vi "Filter And List Controls.vi"(8 "Error In":errorcluster, 10 "Control Refs":refnum<vi>[](array[refnum]), 11 "Control Reference Lists In":T1) -> (0 "Error Out":errorcluster, 3 "Control Reference Lists Out":T1)   [LabVIEW 2021, in "Appearance Actor.lvlib" / "Appearance Actor.lvclass"]
uses:
  Appearance Actor.lvclass
  Typedefs/Control Reference Lists--cluster.ctl
  Typedefs/Control Reference Lists-TitleBar--cluster.ctl
  Typedefs/Control Reference Lists-SideMenu--cluster.ctl
  Typedefs/Control Reference Lists-BodyPane--cluster.ctl
  Typedefs/Control Reference Lists-StatusBar--cluster.ctl
  <vilib>/regexp/Match Regular Expression.xnode
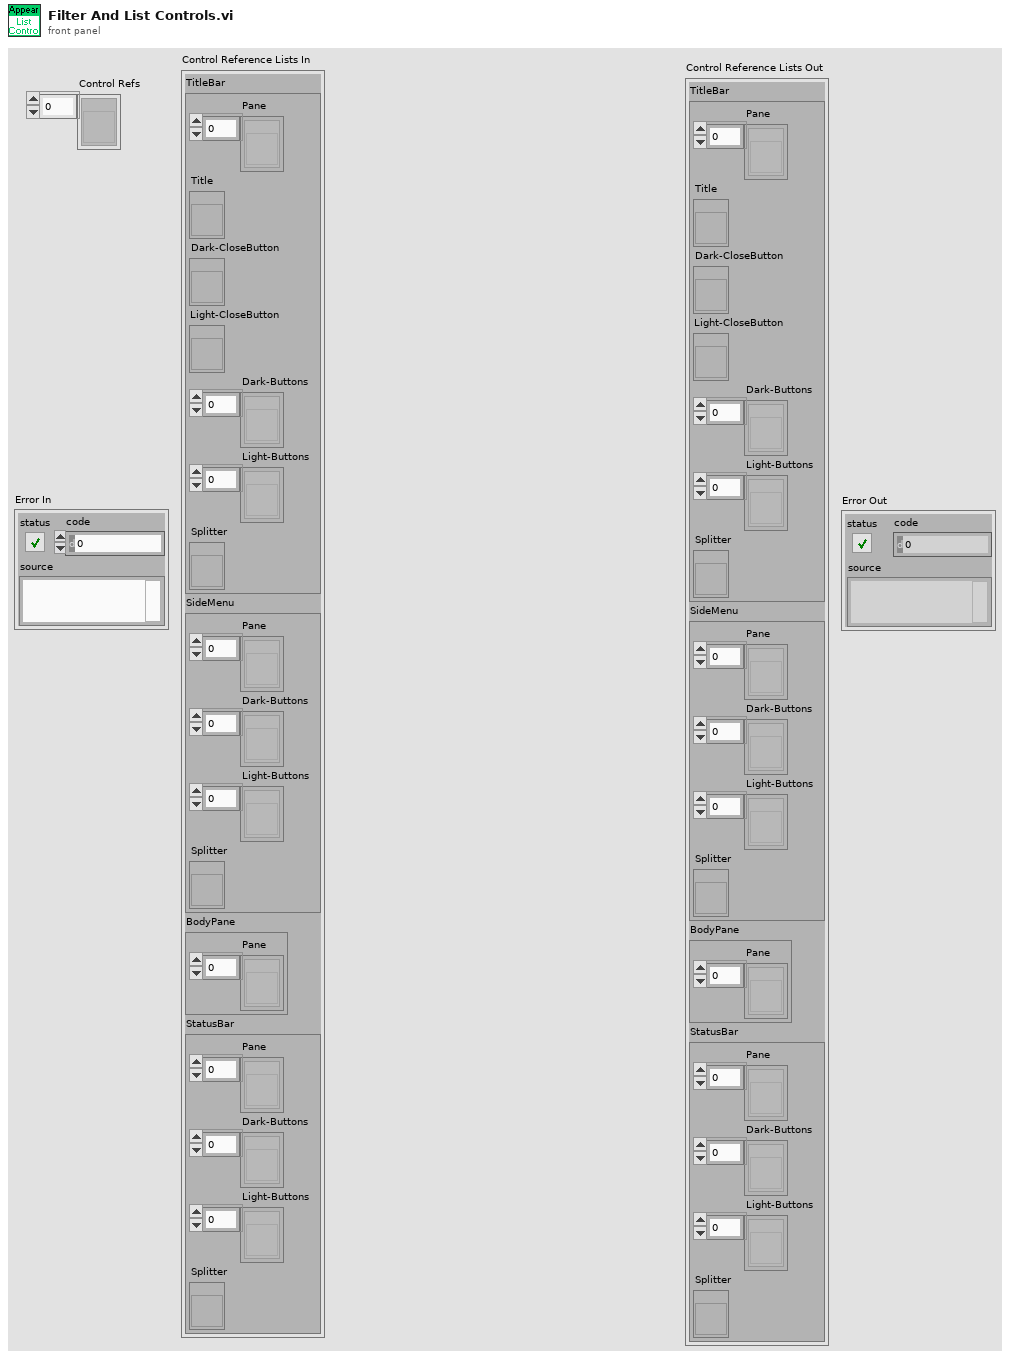
[diagram p1: front panel]
types:
  T1 = typedef "Appearance Actor.lvlib/Appearance Actor.lvclass/Control Reference Lists--cluster.ctl" = cluster{"TitleBar":T2, "SideMenu":T3, "BodyPane":T4, "StatusBar":T5}
  T2 = typedef "Appearance Actor.lvlib/Appearance Actor.lvclass/Control Reference Lists-TitleBar--cluster.ctl" = cluster{"Pane":refnum<vi>[], "Title":refnum<vi>, "Dark-CloseButton":refnum<vi>, "Light-CloseButton":refnum<vi>, "Dark-Buttons":refnum<vi>[], "Light-Buttons":refnum<vi>[], "Splitter":refnum<vi>}
  T3 = typedef "Appearance Actor.lvlib/Appearance Actor.lvclass/Control Reference Lists-SideMenu--cluster.ctl" = cluster{"Pane":refnum<vi>[], "Dark-Buttons":refnum<vi>[], "Light-Buttons":refnum<vi>[], "Splitter":refnum<vi>}
  T4 = typedef "Appearance Actor.lvlib/Appearance Actor.lvclass/Control Reference Lists-BodyPane--cluster.ctl" = cluster{"Pane":refnum<vi>[]}
  T5 = typedef "Appearance Actor.lvlib/Appearance Actor.lvclass/Control Reference Lists-StatusBar--cluster.ctl" = cluster{"Pane":refnum<vi>[], "Dark-Buttons":refnum<vi>[], "Light-Buttons":refnum<vi>[], "Splitter":refnum<vi>}
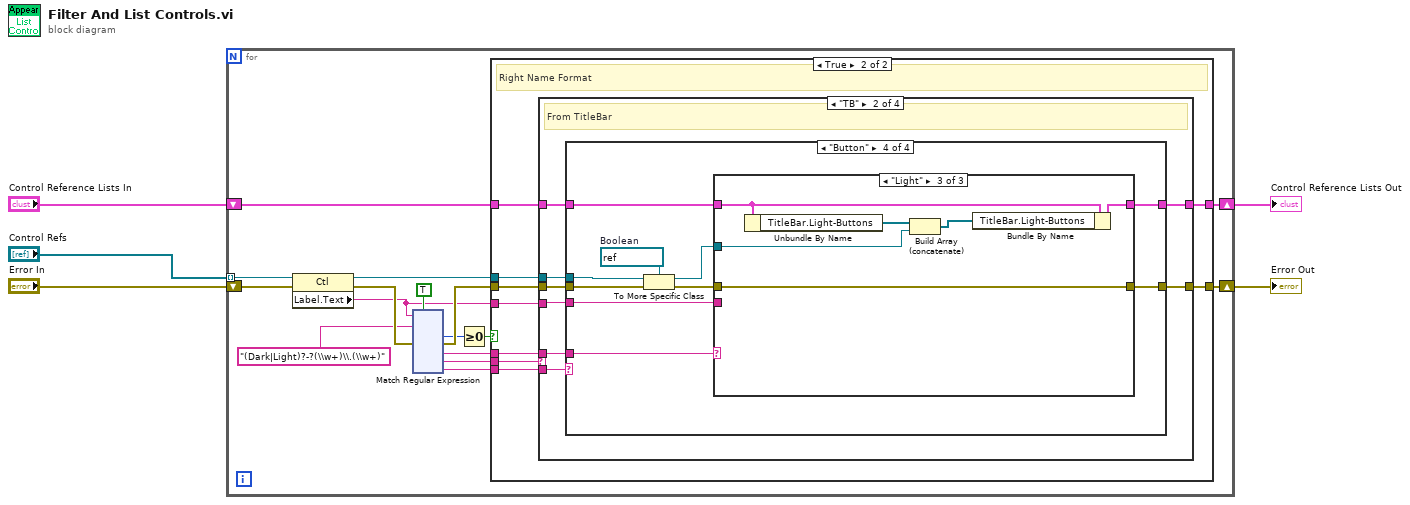
[diagram p0: block diagram]
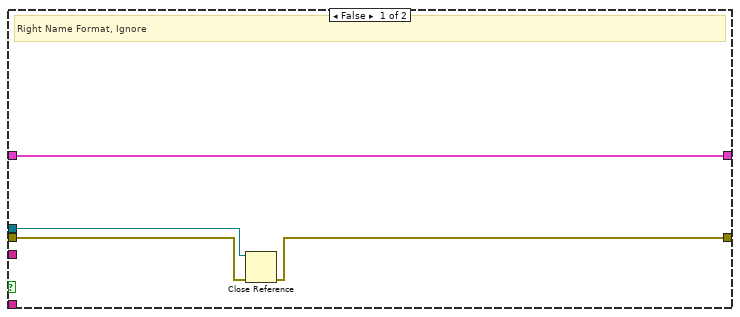
[diagram p2: hidden frame]
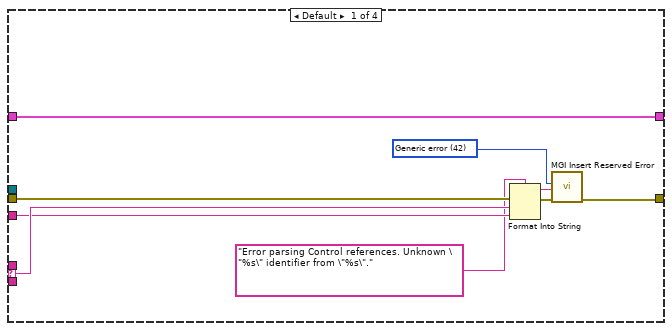
[diagram p3: hidden frame]
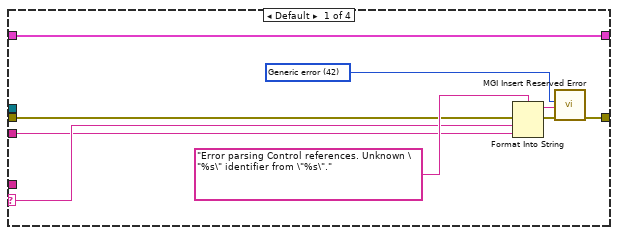
[diagram p4: hidden frame]
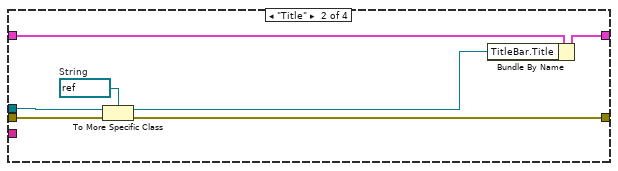
[diagram p5: hidden frame]
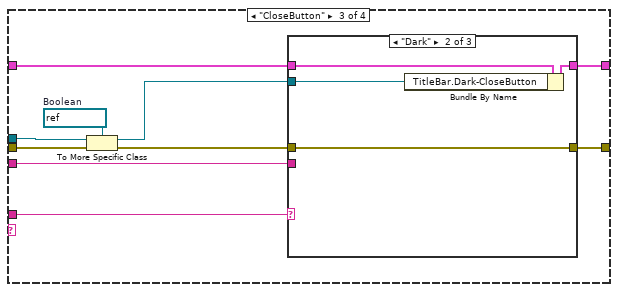
[diagram p6: hidden frame]
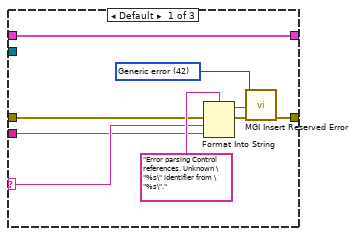
[diagram p7: hidden frame]
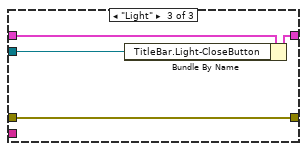
[diagram p8: hidden frame]
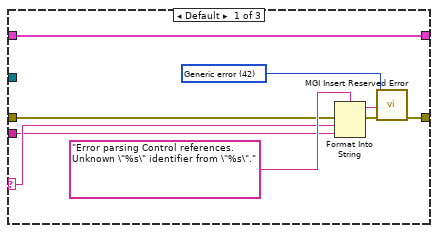
[diagram p9: hidden frame]
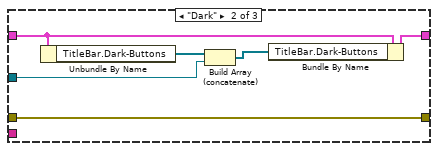
[diagram p10: hidden frame]
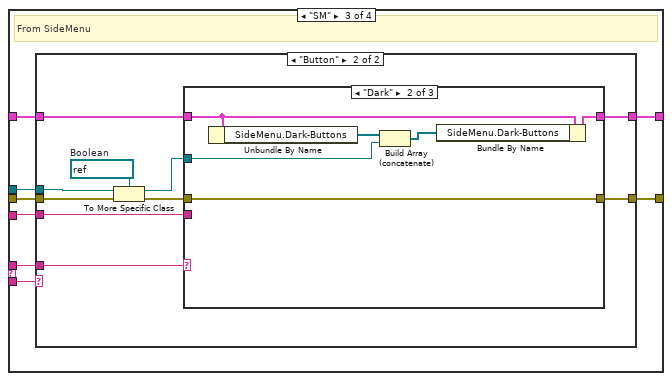
[diagram p11: hidden frame]
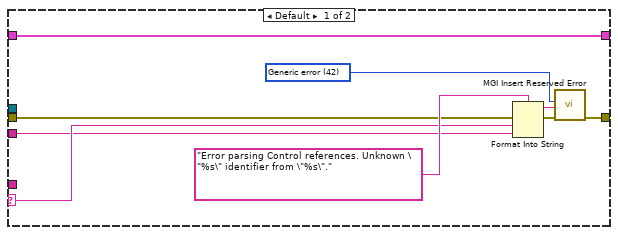
[diagram p12: hidden frame]
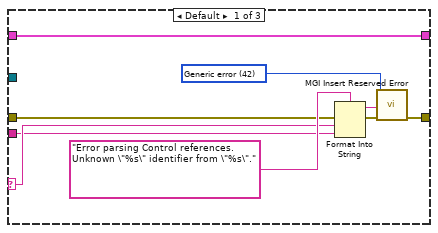
[diagram p13: hidden frame]
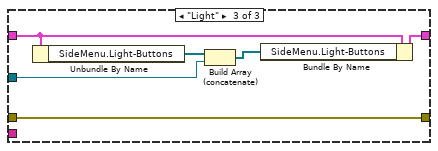
[diagram p14: hidden frame]
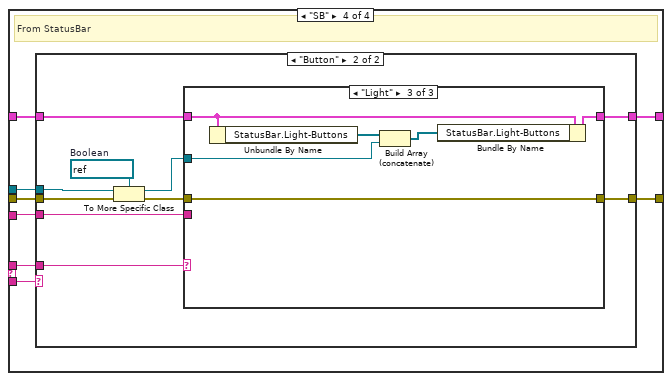
[diagram p15: hidden frame]
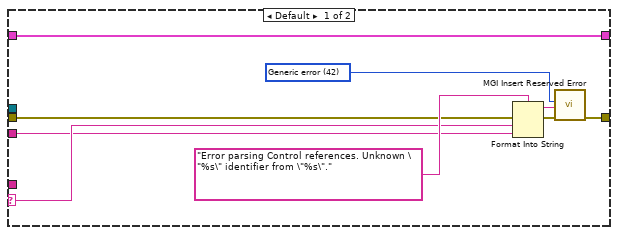
[diagram p16: hidden frame]
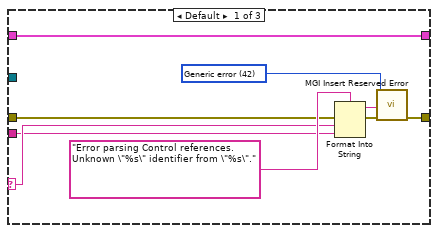
[diagram p17: hidden frame]
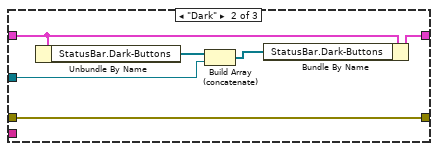
[diagram p18: hidden frame]
diagram:
  n1 = for {
    shift-right: [w9] -> w4
    shift-left: "Control Reference Lists In" -> [w16]
    shift-right: [w14] -> w3
    shift-left: "Error In" -> [w20]
    tunnel: "Control Refs" -> [w21] mode=indexing
    n2 = property class="Ctl"(reference=w21, error in=w20) -> (reference out=w8:refnum<vi>, error out=w19:errorcluster, "Label.Text"=w10:string)
    n3 = xnode "Match Regular Expression"("input string"=w10, "regular expression"="(Dark|Light)?-?(\\w+)\\.(\\w+)", "error in"=w19, "ignore case? (F)"=TRUE) -> ("offset past match"=w7:i32, "error out"=w13:errorcluster, "submatch 1"=w12:string, "submatch 2"=w15:string, "submatch 3"=w11:string)  [unwired: 2 in, 3 out]
    n4 = Greater Or Equal To 0?(x=w7) -> (x >= 0?=w6:bool)
    n5 = case shown="True" w6 {
      tunnel: w16 -> [w25 w34]
      tunnel: w15 -> [_ w33]
      tunnel: [w22 w32] -> w14
      tunnel: w13 -> [w23 w31]
      tunnel: w12 -> [_ w30]
      tunnel: w11 -> [_ w29]
      tunnel: w10 -> [_ w28]
      tunnel: [w25 w27] -> w9
      tunnel: w8 -> [w24 w26]
      frame False {
        # "Right Name Format, Ignore"
        n6 = Close Reference(reference=w24, error in (no error)=w23) -> (error out=w22:errorcluster)
      }
      frame True {
        # "Right Name Format"
        n7 = case shown="\"TB\"" w33 {
          selector: w33 -> [w38 _ _ _]
          tunnel: w34 -> [w36 w47 w129 w177]
          tunnel: [w39 w49 w131 w179] -> w32
          tunnel: w31 -> [w40 w50 w132 w180]
          tunnel: w30 -> [_ w44 w126 w174]
          tunnel: w29 -> [_ w51 w133 w181]
          tunnel: w28 -> [w37 w48 w130 w178]
          tunnel: [w36 w46 w128 w176] -> w27
          tunnel: w26 -> [_ w45 w127 w175]
          frame Default {
            w41 = 42 items=["No error", "Argument error", "Memory is full", "Out of zone", "End of file", "File already open", "Generic file I/O error", "File not found", "File permission error", "Disk is full", "Duplicate path", "Too many files open", "System feature not enabled", "Resource file not found", "Cannot add resource", "Resource not found", "Image not found", "Image memory error", "Pen does not exist", "Config type invalid", "Config token not found", "Config parse error", "Config memory error", "Bad external code format", "Bad external code offset", "External code not present", "Null window", "Destroy window error", "Null menu", "Print aborted", "Bad print record", "Print driver error", "Windows error during printing", "Memory error during printing", "Print dialog error", "Generic print error", "Invalid device refnum", "Device not found", "Device parameter error", "Device unit error", "Cannot open device", "Device call aborted", "Generic error", "Cancelled by user", "Object ID too low", "Object ID too high", "Object not in heap", "Unknown heap", "Unknown object (invalid DefProc)", "Unknown object (DefProc not in table)", "Message out of range", "Invalid (null) method", "Unknown message", "Manager call not supported", "Bad address", "Network operation in progress", "Network operation timed out", "Connection is busy", "Network attribute not supported", "Network error", "Address in use", "System out of memory", "Connection aborted", "Connection refused", "Not connected", "Already connected", "Connection closed", "Initialization error (interapplication manager)", "Bad occurrence", "Wait on unbound occurrence handler", "Occurrence queue overflow", "Datalog type conflict", "Unused", "Unrecognized type (interapplication manager)", "Memory corrupt", "Failed to make temporary DLL", "Old CIN version", "Drag socket not found", "Failed to load drop-object", "Failed to register OLE object", "Failed to release OLE object", "Format specifier type mismatch", "Unknown format specifier", "Too few format specifiers", "Too many format specifiers", "Scan failed", "Newer CIN version", "OLE Convert", "Runtime menu error", "Password tampered", "Unknown error code"] ("Reserved Error Code (Generic error)")
            n8 = Format Into String(format string="Error parsing Control references. Unknown \"%s\" identifier from \"%s\".", error in=w40, w38, w37) -> (resulting string=w43:string, error out=w42:errorcluster)  [unwired: 1 in]
            n9 = call <userlib>:"MGI Insert Reserved Error.vi"("Error In"=w42, "Error Description"=w43, "Reserved Error Code (Generic error)"=w41) -> ("Error Out"=w39:errorcluster)  [unwired: 8 in]
          }
          frame "TB" {
            # "From TitleBar"
            n10 = case shown="\"Button\"" w51 {
              selector: w51 -> [w54 _ _ _]
              tunnel: w50 -> [w56 w62 w72 w99]
              tunnel: [w55 w61 w69 w96] -> w49
              tunnel: w48 -> [w53 _ w68 w95]
              tunnel: w47 -> [w52 w67 w77 w104]
              tunnel: [w52 w66 w76 w103] -> w46
              tunnel: w45 -> [_ w64 w74 w101]
              tunnel: w44 -> [_ _ w71 w98]
              frame Default {
                w58 = 42 items=["No error", "Argument error", "Memory is full", "Out of zone", "End of file", "File already open", "Generic file I/O error", "File not found", "File permission error", "Disk is full", "Duplicate path", "Too many files open", "System feature not enabled", "Resource file not found", "Cannot add resource", "Resource not found", "Image not found", "Image memory error", "Pen does not exist", "Config type invalid", "Config token not found", "Config parse error", "Config memory error", "Bad external code format", "Bad external code offset", "External code not present", "Null window", "Destroy window error", "Null menu", "Print aborted", "Bad print record", "Print driver error", "Windows error during printing", "Memory error during printing", "Print dialog error", "Generic print error", "Invalid device refnum", "Device not found", "Device parameter error", "Device unit error", "Cannot open device", "Device call aborted", "Generic error", "Cancelled by user", "Object ID too low", "Object ID too high", "Object not in heap", "Unknown heap", "Unknown object (invalid DefProc)", "Unknown object (DefProc not in table)", "Message out of range", "Invalid (null) method", "Unknown message", "Manager call not supported", "Bad address", "Network operation in progress", "Network operation timed out", "Connection is busy", "Network attribute not supported", "Network error", "Address in use", "System out of memory", "Connection aborted", "Connection refused", "Not connected", "Already connected", "Connection closed", "Initialization error (interapplication manager)", "Bad occurrence", "Wait on unbound occurrence handler", "Occurrence queue overflow", "Datalog type conflict", "Unused", "Unrecognized type (interapplication manager)", "Memory corrupt", "Failed to make temporary DLL", "Old CIN version", "Drag socket not found", "Failed to load drop-object", "Failed to register OLE object", "Failed to release OLE object", "Format specifier type mismatch", "Unknown format specifier", "Too few format specifiers", "Too many format specifiers", "Scan failed", "Newer CIN version", "OLE Convert", "Runtime menu error", "Password tampered", "Unknown error code"] ("Reserved Error Code (Generic error)")
                n11 = Format Into String(format string="Error parsing Control references. Unknown \"%s\" identifier from \"%s\".", error in=w56, w54, w53) -> (resulting string=w60:string, error out=w59:errorcluster)  [unwired: 1 in]
                n12 = call <userlib>:"MGI Insert Reserved Error.vi"("Error In"=w59, "Error Description"=w60, "Reserved Error Code (Generic error)"=w58) -> ("Error Out"=w55:errorcluster)  [unwired: 8 in]
              }
              frame "Title" {
                w65 = refnum<vi> refnum  # String
                n13 = To More Specific Class(target class=w65, reference=w64, error in=w62) -> (specific class reference=w63:refnum<vi>, error out=w61:errorcluster)
                n14 = Bundle By Name(cluster=w67, "TitleBar.Title"=w63) -> (w66:T1)
              }
              frame "CloseButton" {
                w75 = refnum<vi> refnum  # Boolean
                n15 = To More Specific Class(target class=w75, reference=w74, error in=w72) -> (specific class reference=w73:refnum<vi>, error out=w70:errorcluster)
                n16 = case shown="\"Dark\"" w71 {
                  selector: w71 -> [w79 _ _]
                  tunnel: w77 -> [w80 w90 w94]
                  tunnel: [w80 w89 w93] -> w76
                  tunnel: w73 -> [_ w88 w92]
                  tunnel: w70 -> [w82 w87 w91]
                  tunnel: [w81 w87 w91] -> w69
                  tunnel: w68 -> [w78 _ _]
                  frame Default {
                    w84 = 42 items=["No error", "Argument error", "Memory is full", "Out of zone", "End of file", "File already open", "Generic file I/O error", "File not found", "File permission error", "Disk is full", "Duplicate path", "Too many files open", "System feature not enabled", "Resource file not found", "Cannot add resource", "Resource not found", "Image not found", "Image memory error", "Pen does not exist", "Config type invalid", "Config token not found", "Config parse error", "Config memory error", "Bad external code format", "Bad external code offset", "External code not present", "Null window", "Destroy window error", "Null menu", "Print aborted", "Bad print record", "Print driver error", "Windows error during printing", "Memory error during printing", "Print dialog error", "Generic print error", "Invalid device refnum", "Device not found", "Device parameter error", "Device unit error", "Cannot open device", "Device call aborted", "Generic error", "Cancelled by user", "Object ID too low", "Object ID too high", "Object not in heap", "Unknown heap", "Unknown object (invalid DefProc)", "Unknown object (DefProc not in table)", "Message out of range", "Invalid (null) method", "Unknown message", "Manager call not supported", "Bad address", "Network operation in progress", "Network operation timed out", "Connection is busy", "Network attribute not supported", "Network error", "Address in use", "System out of memory", "Connection aborted", "Connection refused", "Not connected", "Already connected", "Connection closed", "Initialization error (interapplication manager)", "Bad occurrence", "Wait on unbound occurrence handler", "Occurrence queue overflow", "Datalog type conflict", "Unused", "Unrecognized type (interapplication manager)", "Memory corrupt", "Failed to make temporary DLL", "Old CIN version", "Drag socket not found", "Failed to load drop-object", "Failed to register OLE object", "Failed to release OLE object", "Format specifier type mismatch", "Unknown format specifier", "Too few format specifiers", "Too many format specifiers", "Scan failed", "Newer CIN version", "OLE Convert", "Runtime menu error", "Password tampered", "Unknown error code"] ("Reserved Error Code (Generic error)")
                    n17 = Format Into String(format string="Error parsing Control references. Unknown \"%s\" identifier from \"%s\".", error in=w82, w79, w78) -> (resulting string=w86:string, error out=w85:errorcluster)  [unwired: 1 in]
                    n18 = call <userlib>:"MGI Insert Reserved Error.vi"("Error In"=w85, "Error Description"=w86, "Reserved Error Code (Generic error)"=w84) -> ("Error Out"=w81:errorcluster)  [unwired: 8 in]
                  }
                  frame "Dark" {
                    n19 = Bundle By Name(cluster=w90, "TitleBar.Dark-CloseButton"=w88) -> (w89:T1)
                  }
                  frame "Light" {
                    n20 = Bundle By Name(cluster=w94, "TitleBar.Light-CloseButton"=w92) -> (w93:T1)
                  }
                }
              }
              frame "Button" {
                w102 = refnum<vi> refnum  # Boolean
                n21 = To More Specific Class(target class=w102, reference=w101, error in=w99) -> (specific class reference=w100:refnum<vi>, error out=w97:errorcluster)
                n22 = case shown="\"Light\"" w98 {
                  selector: w98 -> [w106 _ _]
                  tunnel: w104 -> [w107 w117 w123]
                  tunnel: [w107 w119 w125] -> w103
                  tunnel: w100 -> [_ w114 w120]
                  tunnel: w97 -> [w109 w118 w124]
                  tunnel: [w108 w118 w124] -> w96
                  tunnel: w95 -> [w105 _ _]
                  frame Default {
                    w111 = 42 items=["No error", "Argument error", "Memory is full", "Out of zone", "End of file", "File already open", "Generic file I/O error", "File not found", "File permission error", "Disk is full", "Duplicate path", "Too many files open", "System feature not enabled", "Resource file not found", "Cannot add resource", "Resource not found", "Image not found", "Image memory error", "Pen does not exist", "Config type invalid", "Config token not found", "Config parse error", "Config memory error", "Bad external code format", "Bad external code offset", "External code not present", "Null window", "Destroy window error", "Null menu", "Print aborted", "Bad print record", "Print driver error", "Windows error during printing", "Memory error during printing", "Print dialog error", "Generic print error", "Invalid device refnum", "Device not found", "Device parameter error", "Device unit error", "Cannot open device", "Device call aborted", "Generic error", "Cancelled by user", "Object ID too low", "Object ID too high", "Object not in heap", "Unknown heap", "Unknown object (invalid DefProc)", "Unknown object (DefProc not in table)", "Message out of range", "Invalid (null) method", "Unknown message", "Manager call not supported", "Bad address", "Network operation in progress", "Network operation timed out", "Connection is busy", "Network attribute not supported", "Network error", "Address in use", "System out of memory", "Connection aborted", "Connection refused", "Not connected", "Already connected", "Connection closed", "Initialization error (interapplication manager)", "Bad occurrence", "Wait on unbound occurrence handler", "Occurrence queue overflow", "Datalog type conflict", "Unused", "Unrecognized type (interapplication manager)", "Memory corrupt", "Failed to make temporary DLL", "Old CIN version", "Drag socket not found", "Failed to load drop-object", "Failed to register OLE object", "Failed to release OLE object", "Format specifier type mismatch", "Unknown format specifier", "Too few format specifiers", "Too many format specifiers", "Scan failed", "Newer CIN version", "OLE Convert", "Runtime menu error", "Password tampered", "Unknown error code"] ("Reserved Error Code (Generic error)")
                    n23 = Format Into String(format string="Error parsing Control references. Unknown \"%s\" identifier from \"%s\".", error in=w109, w106, w105) -> (resulting string=w113:string, error out=w112:errorcluster)  [unwired: 1 in]
                    n24 = call <userlib>:"MGI Insert Reserved Error.vi"("Error In"=w112, "Error Description"=w113, "Reserved Error Code (Generic error)"=w111) -> ("Error Out"=w108:errorcluster)  [unwired: 8 in]
                  }
                  frame "Dark" {
                    n25 = Unbundle By Name(w117) -> ("TitleBar.Dark-Buttons"=w116:refnum<vi>[])
                    n26 = Build Array (concatenate)(w116, w114) -> (w115:refnum<vi>[])
                    n27 = Bundle By Name(cluster=w117, "TitleBar.Dark-Buttons"=w115) -> (w119:T1)
                  }
                  frame "Light" {
                    n28 = Unbundle By Name(w123) -> ("TitleBar.Light-Buttons"=w122:refnum<vi>[])
                    n29 = Build Array (concatenate)(w122, w120) -> (w121:refnum<vi>[])
                    n30 = Bundle By Name(cluster=w123, "TitleBar.Light-Buttons"=w121) -> (w125:T1)
                  }
                }
              }
            }
          }
          frame "SM" {
            # "From SideMenu"
            n31 = case shown="\"Button\"" w133 {
              selector: w133 -> [w136 _]
              tunnel: w132 -> [w138 w147]
              tunnel: [w137 w144] -> w131
              tunnel: w130 -> [w135 w143]
              tunnel: w129 -> [w134 w152]
              tunnel: [w134 w151] -> w128
              tunnel: w127 -> [_ w149]
              tunnel: w126 -> [_ w146]
              frame Default {
                w140 = 42 items=["No error", "Argument error", "Memory is full", "Out of zone", "End of file", "File already open", "Generic file I/O error", "File not found", "File permission error", "Disk is full", "Duplicate path", "Too many files open", "System feature not enabled", "Resource file not found", "Cannot add resource", "Resource not found", "Image not found", "Image memory error", "Pen does not exist", "Config type invalid", "Config token not found", "Config parse error", "Config memory error", "Bad external code format", "Bad external code offset", "External code not present", "Null window", "Destroy window error", "Null menu", "Print aborted", "Bad print record", "Print driver error", "Windows error during printing", "Memory error during printing", "Print dialog error", "Generic print error", "Invalid device refnum", "Device not found", "Device parameter error", "Device unit error", "Cannot open device", "Device call aborted", "Generic error", "Cancelled by user", "Object ID too low", "Object ID too high", "Object not in heap", "Unknown heap", "Unknown object (invalid DefProc)", "Unknown object (DefProc not in table)", "Message out of range", "Invalid (null) method", "Unknown message", "Manager call not supported", "Bad address", "Network operation in progress", "Network operation timed out", "Connection is busy", "Network attribute not supported", "Network error", "Address in use", "System out of memory", "Connection aborted", "Connection refused", "Not connected", "Already connected", "Connection closed", "Initialization error (interapplication manager)", "Bad occurrence", "Wait on unbound occurrence handler", "Occurrence queue overflow", "Datalog type conflict", "Unused", "Unrecognized type (interapplication manager)", "Memory corrupt", "Failed to make temporary DLL", "Old CIN version", "Drag socket not found", "Failed to load drop-object", "Failed to register OLE object", "Failed to release OLE object", "Format specifier type mismatch", "Unknown format specifier", "Too few format specifiers", "Too many format specifiers", "Scan failed", "Newer CIN version", "OLE Convert", "Runtime menu error", "Password tampered", "Unknown error code"] ("Reserved Error Code (Generic error)")
                n32 = Format Into String(format string="Error parsing Control references. Unknown \"%s\" identifier from \"%s\".", error in=w138, w136, w135) -> (resulting string=w142:string, error out=w141:errorcluster)  [unwired: 1 in]
                n33 = call <userlib>:"MGI Insert Reserved Error.vi"("Error In"=w141, "Error Description"=w142, "Reserved Error Code (Generic error)"=w140) -> ("Error Out"=w137:errorcluster)  [unwired: 8 in]
              }
              frame "Button" {
                w150 = refnum<vi> refnum  # Boolean
                n34 = To More Specific Class(target class=w150, reference=w149, error in=w147) -> (specific class reference=w148:refnum<vi>, error out=w145:errorcluster)
                n35 = case shown="\"Dark\"" w146 {
                  selector: w146 -> [w154 _ _]
                  tunnel: w152 -> [w155 w165 w171]
                  tunnel: [w155 w167 w173] -> w151
                  tunnel: w148 -> [_ w162 w168]
                  tunnel: w145 -> [w157 w166 w172]
                  tunnel: [w156 w166 w172] -> w144
                  tunnel: w143 -> [w153 _ _]
                  frame Default {
                    w159 = 42 items=["No error", "Argument error", "Memory is full", "Out of zone", "End of file", "File already open", "Generic file I/O error", "File not found", "File permission error", "Disk is full", "Duplicate path", "Too many files open", "System feature not enabled", "Resource file not found", "Cannot add resource", "Resource not found", "Image not found", "Image memory error", "Pen does not exist", "Config type invalid", "Config token not found", "Config parse error", "Config memory error", "Bad external code format", "Bad external code offset", "External code not present", "Null window", "Destroy window error", "Null menu", "Print aborted", "Bad print record", "Print driver error", "Windows error during printing", "Memory error during printing", "Print dialog error", "Generic print error", "Invalid device refnum", "Device not found", "Device parameter error", "Device unit error", "Cannot open device", "Device call aborted", "Generic error", "Cancelled by user", "Object ID too low", "Object ID too high", "Object not in heap", "Unknown heap", "Unknown object (invalid DefProc)", "Unknown object (DefProc not in table)", "Message out of range", "Invalid (null) method", "Unknown message", "Manager call not supported", "Bad address", "Network operation in progress", "Network operation timed out", "Connection is busy", "Network attribute not supported", "Network error", "Address in use", "System out of memory", "Connection aborted", "Connection refused", "Not connected", "Already connected", "Connection closed", "Initialization error (interapplication manager)", "Bad occurrence", "Wait on unbound occurrence handler", "Occurrence queue overflow", "Datalog type conflict", "Unused", "Unrecognized type (interapplication manager)", "Memory corrupt", "Failed to make temporary DLL", "Old CIN version", "Drag socket not found", "Failed to load drop-object", "Failed to register OLE object", "Failed to release OLE object", "Format specifier type mismatch", "Unknown format specifier", "Too few format specifiers", "Too many format specifiers", "Scan failed", "Newer CIN version", "OLE Convert", "Runtime menu error", "Password tampered", "Unknown error code"] ("Reserved Error Code (Generic error)")
                    n36 = Format Into String(format string="Error parsing Control references. Unknown \"%s\" identifier from \"%s\".", error in=w157, w154, w153) -> (resulting string=w161:string, error out=w160:errorcluster)  [unwired: 1 in]
                    n37 = call <userlib>:"MGI Insert Reserved Error.vi"("Error In"=w160, "Error Description"=w161, "Reserved Error Code (Generic error)"=w159) -> ("Error Out"=w156:errorcluster)  [unwired: 8 in]
                  }
                  frame "Dark" {
                    n38 = Unbundle By Name(w165) -> ("SideMenu.Dark-Buttons"=w164:refnum<vi>[])
                    n39 = Build Array (concatenate)(w164, w162) -> (w163:refnum<vi>[])
                    n40 = Bundle By Name(cluster=w165, "SideMenu.Dark-Buttons"=w163) -> (w167:T1)
                  }
                  frame "Light" {
                    n41 = Unbundle By Name(w171) -> ("SideMenu.Light-Buttons"=w170:refnum<vi>[])
                    n42 = Build Array (concatenate)(w170, w168) -> (w169:refnum<vi>[])
                    n43 = Bundle By Name(cluster=w171, "SideMenu.Light-Buttons"=w169) -> (w173:T1)
                  }
                }
              }
            }
          }
          frame "SB" {
            # "From StatusBar"
            n44 = case shown="\"Button\"" w181 {
              selector: w181 -> [w184 _]
              tunnel: w180 -> [w186 w195]
              tunnel: [w185 w192] -> w179
              tunnel: w178 -> [w183 w191]
              tunnel: w177 -> [w182 w200]
              tunnel: [w182 w199] -> w176
              tunnel: w175 -> [_ w197]
              tunnel: w174 -> [_ w194]
              frame Default {
                w188 = 42 items=["No error", "Argument error", "Memory is full", "Out of zone", "End of file", "File already open", "Generic file I/O error", "File not found", "File permission error", "Disk is full", "Duplicate path", "Too many files open", "System feature not enabled", "Resource file not found", "Cannot add resource", "Resource not found", "Image not found", "Image memory error", "Pen does not exist", "Config type invalid", "Config token not found", "Config parse error", "Config memory error", "Bad external code format", "Bad external code offset", "External code not present", "Null window", "Destroy window error", "Null menu", "Print aborted", "Bad print record", "Print driver error", "Windows error during printing", "Memory error during printing", "Print dialog error", "Generic print error", "Invalid device refnum", "Device not found", "Device parameter error", "Device unit error", "Cannot open device", "Device call aborted", "Generic error", "Cancelled by user", "Object ID too low", "Object ID too high", "Object not in heap", "Unknown heap", "Unknown object (invalid DefProc)", "Unknown object (DefProc not in table)", "Message out of range", "Invalid (null) method", "Unknown message", "Manager call not supported", "Bad address", "Network operation in progress", "Network operation timed out", "Connection is busy", "Network attribute not supported", "Network error", "Address in use", "System out of memory", "Connection aborted", "Connection refused", "Not connected", "Already connected", "Connection closed", "Initialization error (interapplication manager)", "Bad occurrence", "Wait on unbound occurrence handler", "Occurrence queue overflow", "Datalog type conflict", "Unused", "Unrecognized type (interapplication manager)", "Memory corrupt", "Failed to make temporary DLL", "Old CIN version", "Drag socket not found", "Failed to load drop-object", "Failed to register OLE object", "Failed to release OLE object", "Format specifier type mismatch", "Unknown format specifier", "Too few format specifiers", "Too many format specifiers", "Scan failed", "Newer CIN version", "OLE Convert", "Runtime menu error", "Password tampered", "Unknown error code"] ("Reserved Error Code (Generic error)")
                n45 = Format Into String(format string="Error parsing Control references. Unknown \"%s\" identifier from \"%s\".", error in=w186, w184, w183) -> (resulting string=w190:string, error out=w189:errorcluster)  [unwired: 1 in]
                n46 = call <userlib>:"MGI Insert Reserved Error.vi"("Error In"=w189, "Error Description"=w190, "Reserved Error Code (Generic error)"=w188) -> ("Error Out"=w185:errorcluster)  [unwired: 8 in]
              }
              frame "Button" {
                w198 = refnum<vi> refnum  # Boolean
                n47 = To More Specific Class(target class=w198, reference=w197, error in=w195) -> (specific class reference=w196:refnum<vi>, error out=w193:errorcluster)
                n48 = case shown="\"Light\"" w194 {
                  selector: w194 -> [w202 _ _]
                  tunnel: w200 -> [w203 w213 w219]
                  tunnel: [w203 w215 w221] -> w199
                  tunnel: w196 -> [_ w210 w216]
                  tunnel: w193 -> [w205 w214 w220]
                  tunnel: [w204 w214 w220] -> w192
                  tunnel: w191 -> [w201 _ _]
                  frame Default {
                    w207 = 42 items=["No error", "Argument error", "Memory is full", "Out of zone", "End of file", "File already open", "Generic file I/O error", "File not found", "File permission error", "Disk is full", "Duplicate path", "Too many files open", "System feature not enabled", "Resource file not found", "Cannot add resource", "Resource not found", "Image not found", "Image memory error", "Pen does not exist", "Config type invalid", "Config token not found", "Config parse error", "Config memory error", "Bad external code format", "Bad external code offset", "External code not present", "Null window", "Destroy window error", "Null menu", "Print aborted", "Bad print record", "Print driver error", "Windows error during printing", "Memory error during printing", "Print dialog error", "Generic print error", "Invalid device refnum", "Device not found", "Device parameter error", "Device unit error", "Cannot open device", "Device call aborted", "Generic error", "Cancelled by user", "Object ID too low", "Object ID too high", "Object not in heap", "Unknown heap", "Unknown object (invalid DefProc)", "Unknown object (DefProc not in table)", "Message out of range", "Invalid (null) method", "Unknown message", "Manager call not supported", "Bad address", "Network operation in progress", "Network operation timed out", "Connection is busy", "Network attribute not supported", "Network error", "Address in use", "System out of memory", "Connection aborted", "Connection refused", "Not connected", "Already connected", "Connection closed", "Initialization error (interapplication manager)", "Bad occurrence", "Wait on unbound occurrence handler", "Occurrence queue overflow", "Datalog type conflict", "Unused", "Unrecognized type (interapplication manager)", "Memory corrupt", "Failed to make temporary DLL", "Old CIN version", "Drag socket not found", "Failed to load drop-object", "Failed to register OLE object", "Failed to release OLE object", "Format specifier type mismatch", "Unknown format specifier", "Too few format specifiers", "Too many format specifiers", "Scan failed", "Newer CIN version", "OLE Convert", "Runtime menu error", "Password tampered", "Unknown error code"] ("Reserved Error Code (Generic error)")
                    n49 = Format Into String(format string="Error parsing Control references. Unknown \"%s\" identifier from \"%s\".", error in=w205, w202, w201) -> (resulting string=w209:string, error out=w208:errorcluster)  [unwired: 1 in]
                    n50 = call <userlib>:"MGI Insert Reserved Error.vi"("Error In"=w208, "Error Description"=w209, "Reserved Error Code (Generic error)"=w207) -> ("Error Out"=w204:errorcluster)  [unwired: 8 in]
                  }
                  frame "Dark" {
                    n51 = Unbundle By Name(w213) -> ("StatusBar.Dark-Buttons"=w212:refnum<vi>[])
                    n52 = Build Array (concatenate)(w212, w210) -> (w211:refnum<vi>[])
                    n53 = Bundle By Name(cluster=w213, "StatusBar.Dark-Buttons"=w211) -> (w215:T1)
                  }
                  frame "Light" {
                    n54 = Unbundle By Name(w219) -> ("StatusBar.Light-Buttons"=w218:refnum<vi>[])
                    n55 = Build Array (concatenate)(w218, w216) -> (w217:refnum<vi>[])
                    n56 = Bundle By Name(cluster=w219, "StatusBar.Light-Buttons"=w217) -> (w221:T1)
                  }
                }
              }
            }
          }
        }
      }
    }
  }
  "Error Out" <- w3
  "Control Reference Lists Out" <- w4
